vi "initialize.vi"(0 "HGF_DSCCommand in":refnum<class "HGF_DSCCommand.lvclass">, 3 "initializationData":variant, 5 "error in (no error)":errorcluster, 7 "binaryString":string, 8 "I8 Array":i8[](array[numeric]), 9 "prependSize? (T)":bool, 11 "byteOrder (0:big-endian, network order)":T1(ring)) -> (14 "HGF_DSCCommand out":refnum<class "HGF_DSCCommand.lvclass">, 17 "found?":bool, 19 "error out":errorcluster)   [LabVIEW 2012, in "HGF_DSC.lvlib" / "HGF_DSCCommand.lvclass"]
uses:
  HGF_DSCCommand.lvclass
  HGF_SV/HGF_SVCommand/HGF_SVCommand.lvclass
  HGF_DSCCommand.lvclass/HGF_DSCCommand.ctl
panel:
  out "error out 2":errorcluster
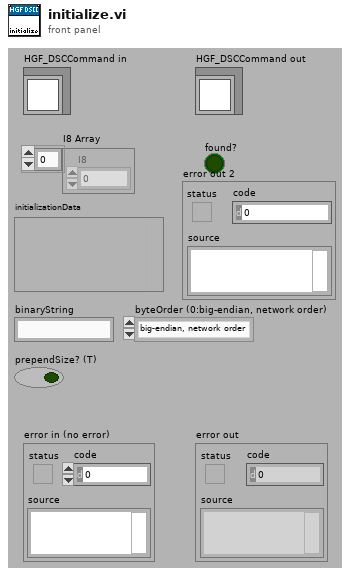
[diagram p1: front panel]
types:
  T1 = enum16{"big-endian, network order", "native, host order", "little-endian"}
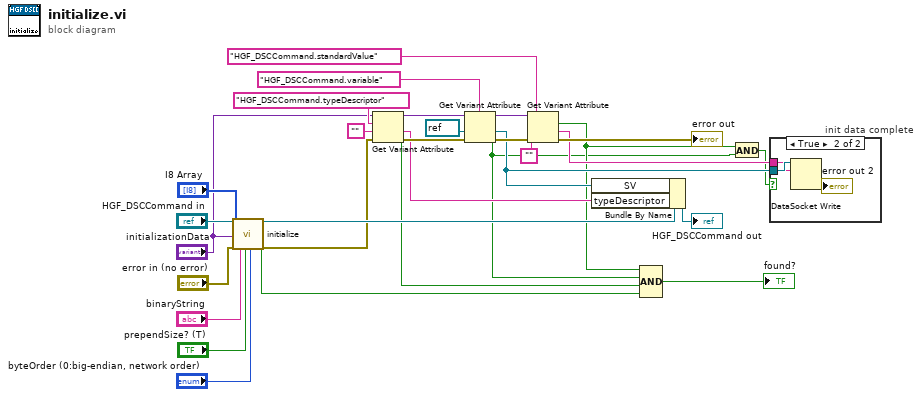
[diagram p0: block diagram]
diagram:
  n1 = call-parent "initialize.vi"("HGF_SVCommand in"="HGF_DSCCommand in", "initializationData"="initializationData", "error in (no error)"="error in (no error)", "binaryString"="binaryString", "I8 Array"="I8 Array", "prependSize? (T)"="prependSize? (T)", "byteOrder (0:big-endian, network order)"="byteOrder (0:big-endian, network order)") -> ("HGF_SVCommand out"=w24:refnum<class "HGF_DSCCommand.lvclass">, "found?"=w14:bool, "error out"=w19:errorcluster)  [unwired: 10 out]
  n2 = Get Variant Attribute(Variant="initializationData", name="HGF_DSCCommand.typeDescriptor", default value (empty Variant)="", error in=w19) -> (duplicate Variant=w17:variant, found=w13:bool, value=w15:string, error out=w18:errorcluster)
  n3 = Get Variant Attribute(Variant=w17, name="HGF_DSCCommand.variable", default value (empty Variant)=refnum<k21> refnum ("Shared Variable"), error in=w18) -> (duplicate Variant=w11:variant, found=w1:bool, value=w6:refnum<k21>, error out=w10:errorcluster)
  n4 = Get Variant Attribute(Variant=w11, name="HGF_DSCCommand.standardValue", default value (empty Variant)="", error in=w10) -> (found=w2:bool, value=w5:string, error out=→"error out":errorcluster)  [unwired: 1 out]
  n5 = Bundle By Name(cluster=w24, "SV"=w6, "typeDescriptor"=w15) -> (→"HGF_DSCCommand out":refnum<class "HGF_DSCCommand.lvclass">)
  n6 = Compound Arithmetic op=AND(w2, w1, w13, w14) -> (→"found?":bool)
  n7 = And(x=w2, y=w1) -> (x .and. y?=w3:bool)
  n8 = case "init data complete" shown="True" w3 {
    tunnel: w6 -> [_ w32]
    tunnel: w5 -> [_ w31]
    frame False {
    }
    frame True {
      n9 = DataSocket Write(10:w31, 11:w32) -> (0:→"error out 2":errorcluster)  [unwired: 1 in, 3 out]
    }
  }
